vi "Measurement.WavelengthSweeping.UI.SetDependencies.vi"(8 "error in (no error)":errorcluster, 10 "Dependencies":T1, 11 "Measurement.WavelengthSweeping.UI in":refnum<class "Measurement.WavelengthSweeping.UI.lvclass">) -> (0 "error out":errorcluster, 3 "Measurement.WavelengthSweeping.UI out":refnum<class "Measurement.WavelengthSweeping.UI.lvclass">)   [LabVIEW 2017, in "Measurement.WavelengthSweeping.UI.lvclass"]
uses:
  Measurement.WavelengthSweeping.UI.lvclass
  Typedefs/Dependencies--Cluster.ctl
  Measurement.WavelengthSweeping/Measurement.WavelengthSweeping.lvclass
  Measurement.WavelengthSweeping.UI.lvclass/Measurement.WavelengthSweeping.UI.ctl
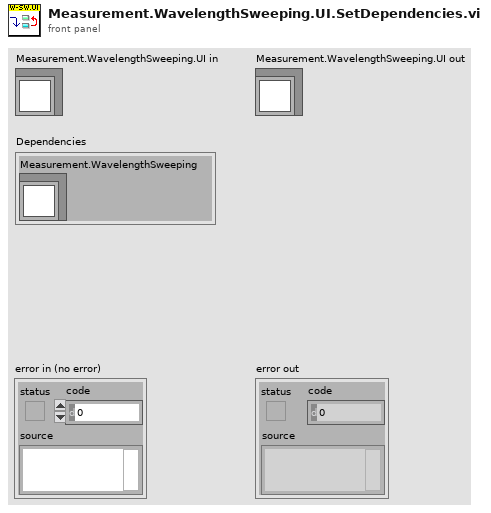
[diagram p1: front panel]
types:
  T1 = typedef "Measurement.WavelengthSweeping.UI.lvclass/Dependencies--Cluster.ctl" = cluster{"Measurement.WavelengthSweeping":refnum<class "Measurement.WavelengthSweeping.lvclass">}
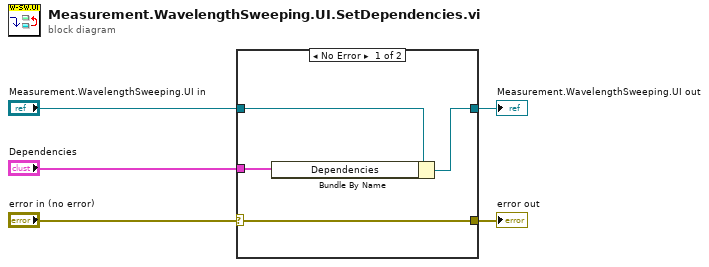
[diagram p0: block diagram]
diagram:
  n1 = case shown="No Error" "error in (no error)" {
    selector: "error in (no error)" -> [w9 w11]
    tunnel: [w9 w11] -> w4
    tunnel: [w6 w10] -> w2
    tunnel: "Measurement.WavelengthSweeping.UI in" -> [w8 w10]
    tunnel: "Dependencies" -> [w7 _]
    frame No Error {
      n2 = Bundle By Name(cluster=w8, "Dependencies"=w7) -> (w6:refnum<class "Measurement.WavelengthSweeping.UI.lvclass">)
    }
    frame Error {
    }
  }
  "error out" <- w4
  "Measurement.WavelengthSweeping.UI out" <- w2
